vi "Read Termination Message.vi"(5 "ignore error on termination message (F)":bool, 8 "timeout (1 ms)":i32=1, 9 "message queue in":T2) -> (2 "termination message":bool, 3 "message queue out":T2, 4 "Message":T1)   [LabVIEW 2014, in "Raspberry Pi Compatible Compiler for LabVIEW.lvlib" / "SimpleMessaging.lvlib"]
doc: "Copyright 2015 National Instruments Corporation\n\n Licensed under the Apache License, Version 2.0 (the \"License\");\n you may not use this file except in compliance with the License.\n You may obtain a copy of the License at\n\n http://www.apache.org/licenses/LICENSE-2.0\n\n Unless required by applicable law or agreed to in writing, software\n distributed under the License is distributed on an \"AS IS\" BASIS,\n WITHOUT WARRANTIES OR CONDITIONS OF ANY KIND, either express or implied.\n See the License for the specific language governing permissions and\n limitations under the License."
uses:
  SimpleMessaging.lvlib
  MessageQueueTD.ctl
  MessageTD.ctl
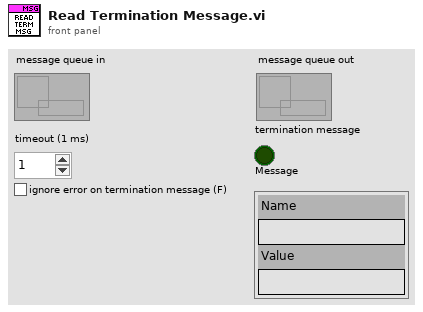
[diagram p1: front panel]
types:
  T1 = typedef "Raspberry Pi Compatible Compiler for LabVIEW.lvlib/SimpleMessaging.lvlib/MessageTD.ctl" = cluster{"Name":string, "Value":string}
  T2 = typedef "Raspberry Pi Compatible Compiler for LabVIEW.lvlib/SimpleMessaging.lvlib/MessageQueueTD.ctl" = refnum<queue>
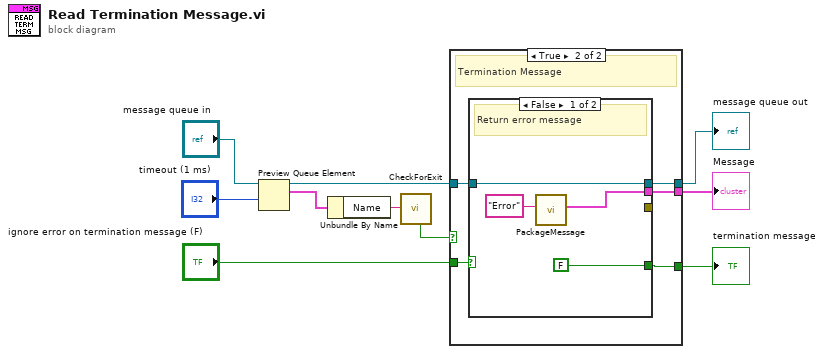
[diagram p0: block diagram]
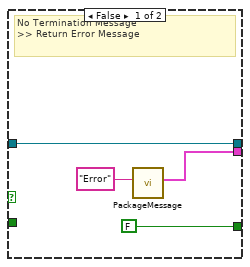
[diagram p2: hidden frame]
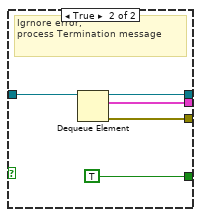
[diagram p3: hidden frame]
diagram:
  n1 = Preview Queue Element(queue="message queue in", timeout in ms (-1)="timeout (1 ms)") -> (queue out=w6:T2, element=w2:T1)  [unwired: 1 in, 2 out]
  n2 = Unbundle By Name(w2) -> ("Name"=w1:string)
  n3 = call "CheckForExit.vi"("Name"=w1) -> ("exit"=w7:bool)  [unwired: 7 in, 1 out]
  n4 = case shown="True" w7 {
    tunnel: [FALSE w17] -> w3
    tunnel: [w13 w16] -> w5
    tunnel: w6 -> [w13 w19]
    tunnel: "ignore error on termination message (F)" -> [_ w18]
    tunnel: [w11 w15] -> w4
    frame False {
      # "No Termination Message\n>> Return Error Message"
      n5 = call "PackageMessage.vi"("Name"="Error") -> ("Message"=w11:T1)  [unwired: 10 in]
    }
    frame True {
      # "Termination Message"
      n6 = case shown="False" w18 {
        tunnel: w19 -> [w22 w28]
        tunnel: [FALSE TRUE] -> w17
        tunnel: [w22 w25] -> w16
        tunnel: [w21 w26] -> w15
        tunnel: [_ w24] -> _
        frame False {
          # "Return error message"
          n7 = call "PackageMessage.vi"("Name"="Error") -> ("Message"=w21:T1)  [unwired: 10 in]
        }
        frame True {
          # "Igrnore error,\nprocess Termination message"
          n8 = Dequeue Element(queue=w28) -> (queue out=w25:T2, element=w26:T1, error out=w24:errorcluster)  [unwired: 2 in, 1 out]
        }
      }
    }
  }
  "message queue out" <- w5
  "Message" <- w4
  "termination message" <- w3
